vi "Get Subpanel Tags and Names.vi"(8 "error in":errorcluster, 10 "subpanel UIDs":i32[](array[numeric]), 11 "VI info in":T1) -> (0 "error out":errorcluster, 1 "subpanel names":string[](array[string]), 2 "subpanel tags":string[](array[string]), 3 "VI info out":T1)   [LabVIEW 2012, in "NI_SE_Config Front Panel Layout.lvlib"]
uses:
  NI_SE_Config Front Panel Layout.lvlib
  VI Info.ctl
  VI Panel Layout/VI Panel Layout.lvclass
  VI Panel Layout/VI Panel Layout.lvclass/VI Panel Layout.ctl
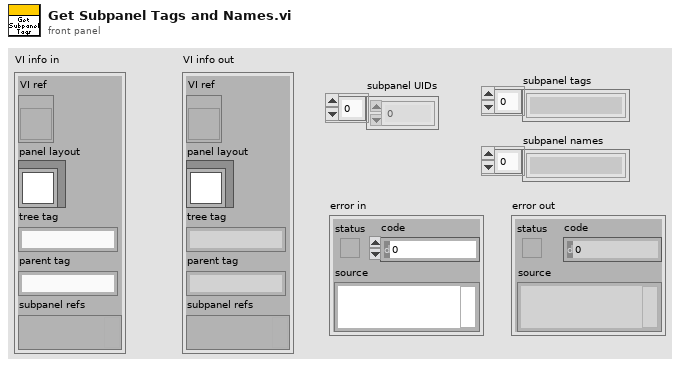
[diagram p1: front panel]
types:
  T1 = typedef "NI_SE_Config Front Panel Layout.lvlib/VI Info.ctl" = cluster{"VI ref":refnum<vi>, "panel layout":refnum<class "VI Panel Layout.lvclass">, "tree tag":string, "parent tag":string, "subpanel refs":variant}
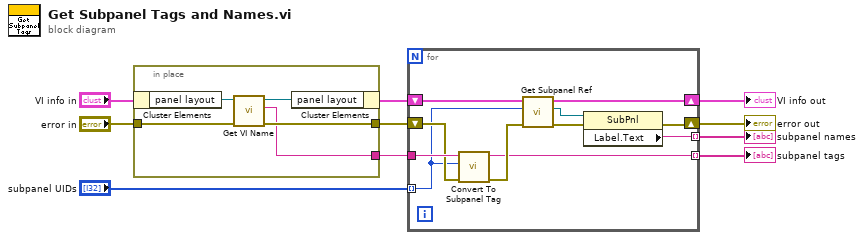
[diagram p0: block diagram]
diagram:
  n1 = in-place {
    in-place-border: "error in" -> [w13]
    in-place-border: [w12] -> w5
    in-place-border: [w11] -> w6
    n2 = in-place-cluster #1("VI info in") -> ("panel layout"=w15:refnum<class "VI Panel Layout.lvclass">)
    n3 = call "Get VI Name.vi"("error in (no error)"=w13, "VI Panel Layout in"=w15) -> ("error out"=w12:errorcluster, "VI name"=w11:string, "VI Panel Layout out"=w14:refnum<class "VI Panel Layout.lvclass">)  [unwired: 7 in]
    n4 = in-place-cluster #1("panel layout"=w14) -> (w8:T1)
  }
  n5 = for {
    shift-right: [w19] -> w4
    shift-left: w8 -> [w23]
    tunnel: "subpanel UIDs" -> [w21] mode=indexing
    tunnel: w6 -> [w26]
    shift-right: [w18] -> w3
    shift-left: w5 -> [w25]
    tunnel: [w17] -> w2 mode=indexing
    tunnel: [w16] -> w1 mode=indexing
    n6 = call "Convert To Subpanel Tag.vi"("error in"=w25, "subpanel UID"=w21, "owning VI name"=w26) -> ("error out"=w22:errorcluster, "subpanel tag"=w16:string)  [unwired: 7 in]
    n7 = call "Get Subpanel Ref.vi"("error in"=w22, "subpanel UID"=w21, "VI info in"=w23) -> ("error out"=w24:errorcluster, "subpanel ref"=w20:refnum<vi>, "VI info out"=w19:T1)  [unwired: 5 in, 1 out]
    n8 = property class="SubPnl"(reference=w20, error in=w24) -> (error out=w18:errorcluster, "Label.Text"=w17:string)  [unwired: 1 out]
  }
  "VI info out" <- w4
  "error out" <- w3
  "subpanel names" <- w2
  "subpanel tags" <- w1
